vi "CheckHeadEnabled.vi"(10 "PrinterInitialization.HIBEnable.#attributes":bool[](array[boolean]), 11 "reordered array":bool[](array[boolean])) -> (3 "Array":bool[](array[boolean]))   [LabVIEW 2022 SP3, in "TopLevel.lvclass"]
uses:
  TopLevel.lvclass
  TopLevel.lvclass/TopLevel.ctl
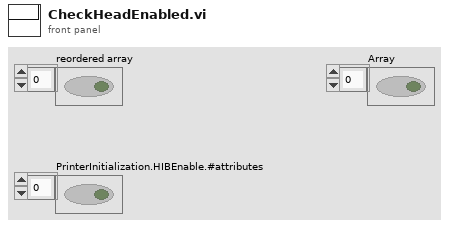
[diagram p1: front panel]
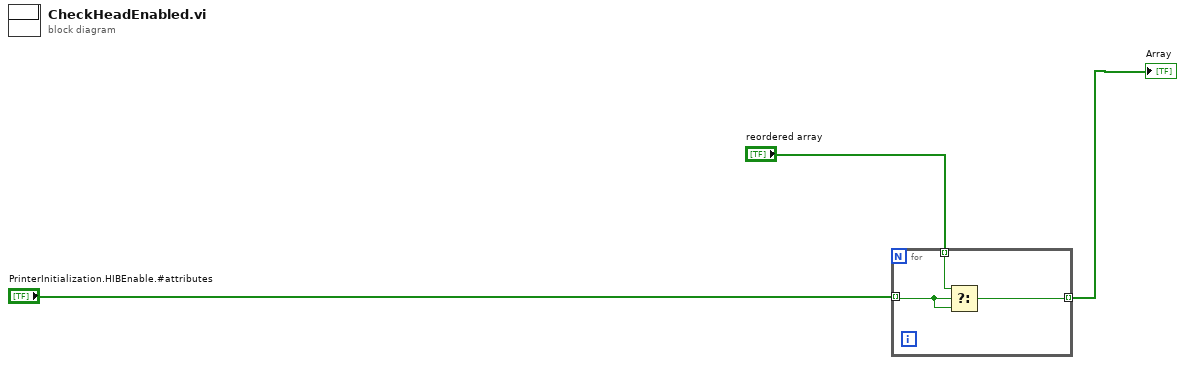
[diagram p0: block diagram]
diagram:
  n1 = for {
    tunnel: "PrinterInitialization.HIBEnable.#attributes" -> [w5] mode=indexing
    tunnel: "reordered array" -> [w6] mode=indexing
    tunnel: [w4] -> w3 mode=indexing
    n2 = Select(t=w6, s=w5, f=w5) -> (s? t:f=w4:bool)
  }
  "Array" <- w3
